vi "Motor controller.vi"(0 "Conveyer Belt":dbl, 1 "Roller":dbl, 2 "Cannon":dbl, 3 "Transfer":dbl, 4 "Flipper":dbl, 5 "Feeder":dbl, 6 "zAvit":dbl, 7 "Camera Servo Y":dbl, 8 "Camera Servo X":dbl, 9 "Canenet":dbl, 10 "Climb Telescopic":dbl) -> ()   [LabVIEW 2012]
uses:
  BotStatus.vi
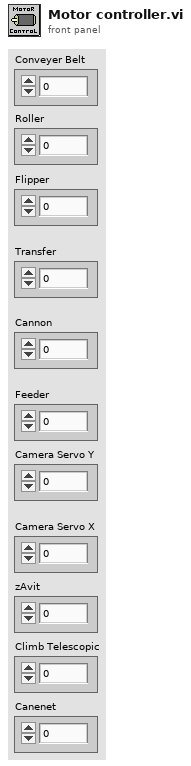
[diagram p1: front panel]
types:
  T1 = typedef "WPI_MotorControlDeviceRef.ctl" = cluster{"DeviceStatus":errorcluster, "Type":enum16{"PWM", "CAN"}, "PWM":cluster{"Digital Module":T2, "PWM Channel":T3, "DeadBand":T4}, "CAN":cluster{"Device Number":u8, "Control Mode":T5, "Semaphore":T6, "Max Vout":dbl}, "Invert":bool, "TransformRef":T7, "InvTransformRef":T7}
  T2 = typedef "FPGA_TypedefDigitalModule.ctl" = enum16{"Digital Module 1", "Digital Module 2"}
  T3 = typedef "FPGA_DIOPWMChannel.ctl" = enum8{"PWM 1", "PWM 2", "PWM 3", "PWM 4", "PWM 5", "PWM 6", "PWM 7", "PWM 8", "PWM 9", "PWM 10", "Invalid"}
  T4 = typedef "WPI_PWMDeadband.ctl" = cluster{"Name":string, "maxPositivePwm":i32, "minPositivePwm":i32, "centerPwm":i32, "maxNegativePwm":i32, "minNegativePwm":i32, "angularRange":u16}
  T5 = typedef "WPI_CANJaguar_ControlMode.ctl" = enum8{"Percent VBus", "Current", "Speed", "Position", "Voltage"}
  T6 = typedef "Semaphore RefNum" = refnum<k1>
  T7 = typedef "WPI_PWMTransform_ConPane.ctl" = refnum<vi>
  T8 = typedef "WPI_ServoDeviceRef.ctl" = cluster{"DeviceStatus":errorcluster, "Digital Module":T2, "PWM Channel":T3, "DeadBand":T4}
  T9 = typedef "WPI_RelayDevRef.ctl" = cluster{"DevStatus":errorcluster, "Relay Channel":T10, "Digital Module":T2, "Relay Direction":T11}
  T10 = typedef "FPGA_DIORelayChannel.ctl" = enum8{"Relay 1", "Relay 2", "Relay 3", "Relay 4", "Relay 5", "Relay 6", "Relay 7", "Relay 8", "Invalid"}
  T11 = typedef "WPI_RelayDirection.ctl" = enum16{"Both directions", "Forward only", "Reverse only"}
  T12 = typedef "WPI_RelayValue.ctl" = enum16{"Off", "On", "Forward", "Reverse"}
  T13 = cluster{"Cannon Upper LS":bool, "Cannon Lower LS":bool}
  T14 = typedef "WPI_DigitalInputDevRef.ctl" = cluster{"DevStatus":errorcluster, "DIO Channel":T15, "Digital Module":T2}
  T15 = typedef "FPGA_DIOChannel.ctl" = enum8{"DIO 1", "DIO 2", "DIO 3", "DIO 4", "DIO 5", "DIO 6", "DIO 7", "DIO 8", "DIO 9", "DIO 10", "DIO 11", "DIO 12", "DIO 13", "DIO 14", "Invalid"}
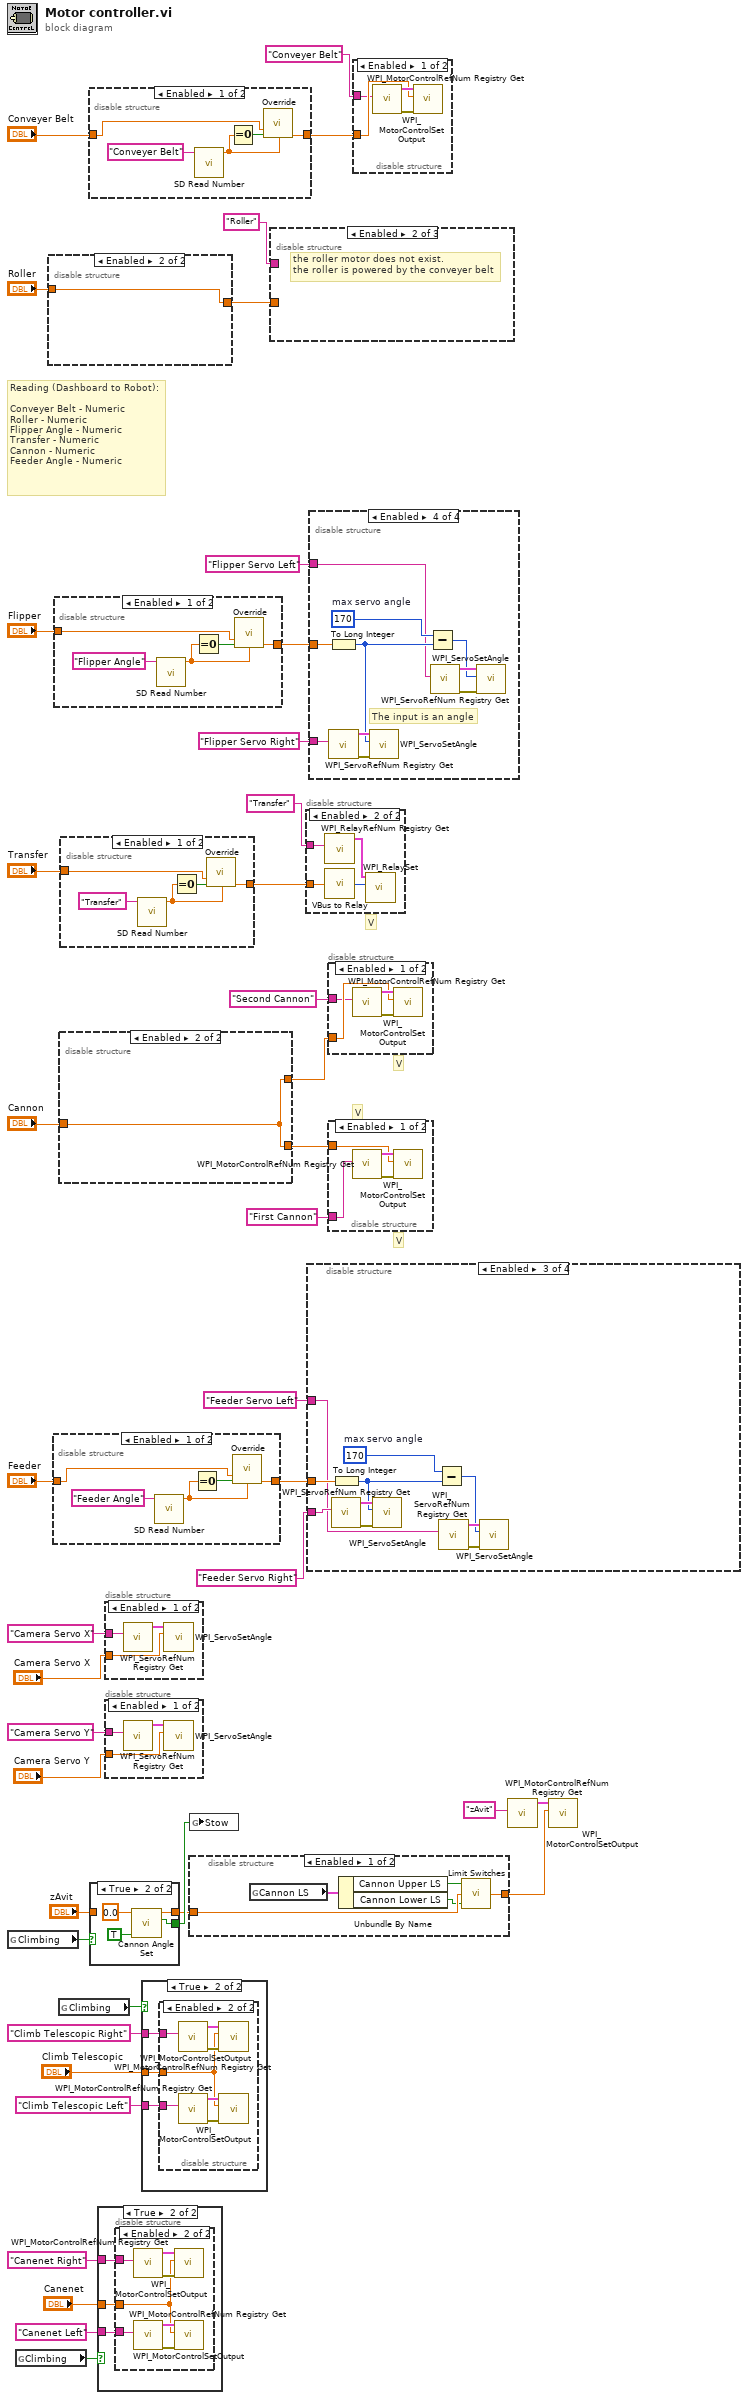
[diagram p0: block diagram]
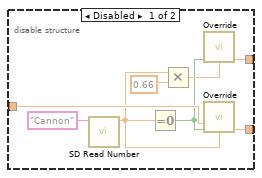
[diagram p5: hidden frame]
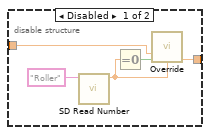
[diagram p8: hidden frame]
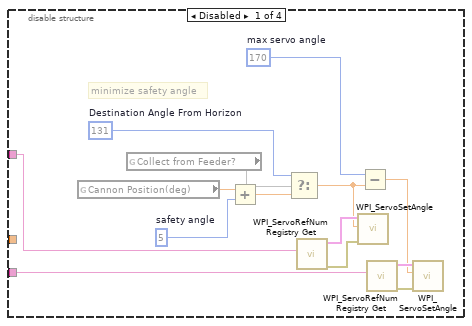
[diagram p11: hidden frame]
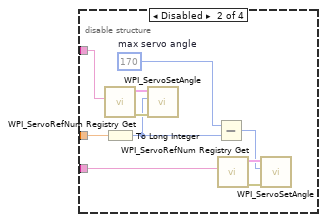
[diagram p12: hidden frame]
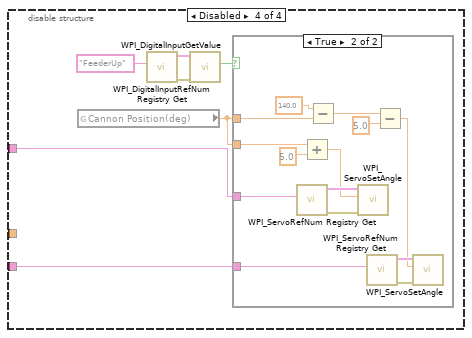
[diagram p13: hidden frame]
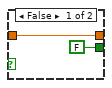
[diagram p15: hidden frame]
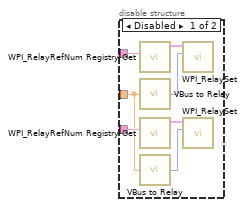
[diagram p19: hidden frame]
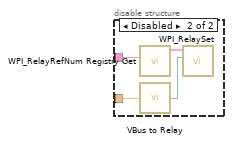
[diagram p20: hidden frame]
diagram:
  # "Reading (Dashboard to Robot):\n\nConveyer Belt - Numeric\nRoller - Numeric\nFlipper Angle - Numeric\nTransfer - Numeric\nCannon - Numeric\nFeeder Angle - Numeric"
  # "V"
  # "V"
  # "V"
  # "V"
  n1 = global read "BotStatus.vi" "Climbing"() -> (w27:bool)
  n2 = global read "BotStatus.vi" "Climbing"() -> (w28:bool)
  n3 = disable-structure shown="Enabled" {
    disable-tunnel: "Roller" -> [w43 w47]
    disable-tunnel: [w42 w47] -> w20
    frame Disabled {
      n4 = call <vilib>:"SD Read Number.vi"("Name"="Roller") -> ("Numeric"=w45:dbl)  [unwired: 8 in, 2 out]
      n5 = Equal To 0?(x=w45) -> (x = 0?=w46:bool)
      n6 = call "Override.vi"("Regualer"=w43, "Override"=w46, "Overriden"=w45) -> ("Output"=w42:dbl)  [unwired: 12 in]
    }
    frame Enabled {
    }
  }
  n7 = disable-structure shown="Enabled" {
    disable-tunnel: [w49 w53] -> w15
    disable-tunnel: "Feeder" -> [w48 w53]
    frame Enabled {
      n8 = call <vilib>:"SD Read Number.vi"("Name"="Feeder Angle") -> ("Numeric"=w52:dbl)  [unwired: 8 in, 2 out]
      n9 = Equal To 0?(x=w52) -> (x = 0?=w51:bool)
      n10 = call "Override.vi"("Regualer"=w48, "Override"=w51, "Overriden"=w52) -> ("Output"=w49:dbl)  [unwired: 12 in]
    }
    frame Disabled {
    }
  }
  n11 = disable-structure shown="Enabled" {
    disable-tunnel: "Flipper" -> [w55 w59]
    disable-tunnel: [w54 w59] -> w19
    frame Enabled {
      n12 = call <vilib>:"SD Read Number.vi"("Name"="Flipper Angle") -> ("Numeric"=w57:dbl)  [unwired: 8 in, 2 out]
      n13 = Equal To 0?(x=w57) -> (x = 0?=w56:bool)
      n14 = call "Override.vi"("Regualer"=w55, "Override"=w56, "Overriden"=w57) -> ("Output"=w54:dbl)  [unwired: 12 in]
    }
    frame Disabled {
    }
  }
  n15 = global read "BotStatus.vi" "Climbing"() -> (w33:bool)
  n16 = disable-structure shown="Enabled" {
    disable-tunnel: "Cannon" -> [w66 w68]
    disable-tunnel: [w65 w68] -> w17
    disable-tunnel: [w60 w68] -> w16
    frame Disabled {
      n17 = call <vilib>:"SD Read Number.vi"("Name"="Cannon") -> ("Numeric"=w63:dbl)  [unwired: 8 in, 2 out]
      n18 = Equal To 0?(x=w63) -> (x = 0?=w64:bool)
      n19 = Multiply(x=w63, y=0.66) -> (x*y=w62:dbl)
      n20 = call "Override.vi"("Override"=w64, "Overriden"=w62) -> ("Output"=w60:dbl)  [unwired: 13 in]
      n21 = call "Override.vi"("Regualer"=w66, "Override"=w64, "Overriden"=w63) -> ("Output"=w65:dbl)  [unwired: 12 in]
    }
    frame Enabled {
    }
  }
  n22 = disable-structure shown="Enabled" {
    disable-tunnel: "Transfer" -> [w70 w74]
    disable-tunnel: [w69 w74] -> w18
    frame Enabled {
      n23 = call <vilib>:"SD Read Number.vi"("Name"="Transfer") -> ("Numeric"=w72:dbl)  [unwired: 8 in, 2 out]
      n24 = Equal To 0?(x=w72) -> (x = 0?=w71:bool)
      n25 = call "Override.vi"("Regualer"=w70, "Override"=w71, "Overriden"=w72) -> ("Output"=w69:dbl)  [unwired: 12 in]
    }
    frame Disabled {
    }
  }
  n26 = disable-structure shown="Enabled" {
    disable-tunnel: [w79 w80] -> w21
    disable-tunnel: "Conveyer Belt" -> [w76 w80]
    frame Enabled {
      n27 = call <vilib>:"SD Read Number.vi"("Name"="Conveyer Belt") -> ("Numeric"=w77:dbl)  [unwired: 8 in, 2 out]
      n28 = Equal To 0?(x=w77) -> (x = 0?=w75:bool)
      n29 = call "Override.vi"("Regualer"=w76, "Override"=w75, "Overriden"=w77) -> ("Output"=w79:dbl)  [unwired: 12 in]
    }
    frame Disabled {
    }
  }
  n30 = case shown="True" w27 {
    tunnel: [w82 w84] -> w14
    tunnel: "zAvit" -> [w82 _]
    tunnel: [FALSE ("On Target") w83] -> w23
    frame False {
    }
    frame True {
      n31 = call "Cannon Angle Set.vi"("set angle 0 to be min angle"=TRUE, "Angle Set Point"=0.0) -> ("On Target"=w83:bool, "zAvit Vbus Out"=w84:dbl)  [unwired: 8 in]
    }
  }
  n32 = case shown="True" w28 {
    tunnel: "Canenet" -> [_ w89]
    tunnel: "Canenet Right" ("refnum name") -> [_ w88]
    tunnel: "Canenet Left" ("refnum name") -> [_ w87]
    frame False {
    }
    frame True {
      n33 = disable-structure shown="Enabled" {
        disable-tunnel: w89 -> [_ w90]
        disable-tunnel: w88 -> [_ w92]
        disable-tunnel: w87 -> [_ w91]
        frame Disabled {
        }
        frame Enabled {
          n34 = call <vilib>:"WPI_MotorControlRefNum Registry Get.vi"("refnum name"=w92) -> ("error out"=w96:errorcluster, "MotorControlDevRef"=w95:T1)  [unwired: 9 in]
          n35 = call <vilib>:"WPI_MotorControlRefNum Registry Get.vi"("refnum name"=w91) -> ("error out"=w93:errorcluster, "MotorControlDevRef"=w94:T1)  [unwired: 9 in]
          n36 = call <vilib>:"WPI_MotorControlSetOutput.vi"("error in (no error)"=w96, "Output"=w90, "MotorControlDevRef"=w95) -> ()  [unwired: 6 in, 3 out]
          n37 = call <vilib>:"WPI_MotorControlSetOutput.vi"("error in (no error)"=w93, "Output"=w90, "MotorControlDevRef"=w94) -> ()  [unwired: 6 in, 3 out]
        }
      }
    }
  }
  n38 = disable-structure shown="Enabled" {
    disable-tunnel: "Camera Servo X" ("refnum name") -> [w99 _]
    disable-tunnel: "Camera Servo X" -> [w97 _]
    frame Enabled {
      n39 = call <vilib>:"WPI_ServoRefNum Registry Get.vi"("refnum name"=w99) -> ("ServoDeviceRef"=w98:T8)  [unwired: 9 in, 1 out]
      n40 = call <vilib>:"WPI_ServoSetAngle.vi"("Angle"=w97, "ServoDeviceRef"=w98) -> ()  [unwired: 8 in, 2 out]
    }
    frame Disabled {
    }
  }
  n41 = disable-structure shown="Enabled" {
    disable-tunnel: "Camera Servo Y" ("refnum name") -> [w102 _]
    disable-tunnel: "Camera Servo Y" -> [w100 _]
    frame Enabled {
      n42 = call <vilib>:"WPI_ServoRefNum Registry Get.vi"("refnum name"=w102) -> ("ServoDeviceRef"=w101:T8)  [unwired: 9 in, 1 out]
      n43 = call <vilib>:"WPI_ServoSetAngle.vi"("Angle"=w100, "ServoDeviceRef"=w101) -> ()  [unwired: 8 in, 2 out]
    }
    frame Disabled {
    }
  }
  n44 = case shown="True" w33 {
    tunnel: "Climb Telescopic" -> [_ w105]
    tunnel: "Climb Telescopic Right" ("refnum name") -> [_ w104]
    tunnel: "Climb Telescopic Left" ("refnum name") -> [_ w103]
    frame False {
    }
    frame True {
      n45 = disable-structure shown="Enabled" {
        disable-tunnel: w105 -> [w107 w113]
        disable-tunnel: w104 -> [w108 w115]
        disable-tunnel: w103 -> [w109 w114]
        frame Disabled {
          n46 = call <vilib>:"WPI_RelayRefNum Registry Get.vi"("refnum name"=w108) -> ("RelayDevRef"=w106:T9)  [unwired: 9 in, 1 out]
          n47 = call "VBus to Relay.vi"("Motor VBus"=w107) -> ("RelayValue"=w112:T12)  [unwired: 3 in]
          n48 = call <vilib>:"WPI_RelayRefNum Registry Get.vi"("refnum name"=w109) -> ("RelayDevRef"=w111:T9)  [unwired: 9 in, 1 out]
          n49 = call "VBus to Relay.vi"("Motor VBus"=w107) -> ("RelayValue"=w110:T12)  [unwired: 3 in]
          n50 = call <vilib>:"WPI_RelaySet.vi"("RelayValue"=w112, "RelayDevRef"=w106) -> ()  [unwired: 8 in, 2 out]
          n51 = call <vilib>:"WPI_RelaySet.vi"("RelayValue"=w110, "RelayDevRef"=w111) -> ()  [unwired: 8 in, 2 out]
        }
        frame Enabled {
          n52 = call <vilib>:"WPI_MotorControlRefNum Registry Get.vi"("refnum name"=w115) -> ("error out"=w119:errorcluster, "MotorControlDevRef"=w118:T1)  [unwired: 9 in]
          n53 = call <vilib>:"WPI_MotorControlRefNum Registry Get.vi"("refnum name"=w114) -> ("error out"=w116:errorcluster, "MotorControlDevRef"=w117:T1)  [unwired: 9 in]
          n54 = call <vilib>:"WPI_MotorControlSetOutput.vi"("error in (no error)"=w119, "Output"=w113, "MotorControlDevRef"=w118) -> ()  [unwired: 6 in, 3 out]
          n55 = call <vilib>:"WPI_MotorControlSetOutput.vi"("error in (no error)"=w116, "Output"=w113, "MotorControlDevRef"=w117) -> ()  [unwired: 6 in, 3 out]
        }
      }
    }
  }
  n56 = global write "BotStatus.vi" "Stow"(w23) -> ()
  n57 = disable-structure shown="Enabled" {
    disable-tunnel: w14 -> [w123 w125]
    disable-tunnel: [w124 w125] -> w13
    frame Enabled {
      n58 = global read "BotStatus.vi" "Cannon LS"() -> (w122:T13)
      n59 = Unbundle By Name(w122) -> ("Cannon Upper LS"=w121:bool, "Cannon Lower LS"=w120:bool)
      n60 = call "Limit Switches.vi"("Backward Limit Switch"=w120, "VBus in"=w123, "Forward Limit Switch"=w121) -> ("VBus out"=w124:dbl)
    }
    frame Disabled {
    }
  }
  n61 = disable-structure shown="Enabled" {
    disable-tunnel: w20 -> [w127 _ w130]
    disable-tunnel: "Roller" ("refnum name") -> [w126 _ w132]
    frame Disabled {
      n62 = call <vilib>:"WPI_MotorControlRefNum Registry Get.vi"("refnum name"=w126) -> ("error out"=w129:errorcluster, "MotorControlDevRef"=w128:T1)  [unwired: 9 in]
      n63 = call <vilib>:"WPI_MotorControlSetOutput.vi"("error in (no error)"=w129, "Output"=w127, "MotorControlDevRef"=w128) -> ()  [unwired: 6 in, 3 out]
    }
    frame Enabled {
      # "the roller motor does not exist.\nthe roller is powered by the conveyer belt"
    }
    frame Disabled {
      n64 = call <vilib>:"WPI_RelayRefNum Registry Get.vi"("refnum name"=w132) -> ("RelayDevRef"=w131:T9)  [unwired: 9 in, 1 out]
      n65 = call "VBus to Relay.vi"("Motor VBus"=w130) -> ("RelayValue"=w133:T12)  [unwired: 3 in]
      n66 = call <vilib>:"WPI_RelaySet.vi"("RelayValue"=w133, "RelayDevRef"=w131) -> ()  [unwired: 8 in, 2 out]
    }
  }
  n67 = disable-structure shown="Enabled" {
    disable-tunnel: w18 -> [w135 w138]
    disable-tunnel: "Transfer" ("refnum name") -> [w134 w140]
    frame Disabled {
      n68 = call <vilib>:"WPI_MotorControlRefNum Registry Get.vi"("refnum name"=w134) -> ("error out"=w137:errorcluster, "MotorControlDevRef"=w136:T1)  [unwired: 9 in]
      n69 = call <vilib>:"WPI_MotorControlSetOutput.vi"("error in (no error)"=w137, "Output"=w135, "MotorControlDevRef"=w136) -> ()  [unwired: 6 in, 3 out]
    }
    frame Enabled {
      n70 = call <vilib>:"WPI_RelayRefNum Registry Get.vi"("refnum name"=w140) -> ("RelayDevRef"=w139:T9)  [unwired: 9 in, 1 out]
      n71 = call "VBus to Relay.vi"("Motor VBus"=w138) -> ("RelayValue"=w141:T12)  [unwired: 3 in]
      n72 = call <vilib>:"WPI_RelaySet.vi"("RelayValue"=w141, "RelayDevRef"=w139) -> ()  [unwired: 8 in, 2 out]
    }
  }
  n73 = disable-structure shown="Enabled" {
    disable-tunnel: "Feeder Servo Left" ("refnum name") -> [w152 w157 w166 w178]
    disable-tunnel: "Feeder Servo Right" ("refnum name") -> [w149 w156 w167 w177]
    disable-tunnel: w15 -> [_ w159 w169 _]
    frame Disabled {
      w144 = 131  # Destination Angle From Horizon
      w148 = 170  # max servo angle
      w153 = 5  # safety angle
      # "minimize safety angle"
      n74 = global read "BotStatus.vi" "Cannon Position(deg)"() -> (w142:dbl)
      n75 = global read "BotStatus.vi" "Collect from Feeder?"() -> (w143)
      n76 = Add(x=w142, y=w153) -> (x+y=w145:dbl)
      n77 = Select(t=w144, s=w143, f=w145) -> (s? t:f=w146:dbl)
      n78 = call <vilib>:"WPI_ServoRefNum Registry Get.vi"("refnum name"=w152) -> ("error out"=w154:errorcluster, "ServoDeviceRef"=w155:T8)  [unwired: 9 in]
      n79 = call <vilib>:"WPI_ServoSetAngle.vi"("error in (no error)"=w154, "Angle"=w146, "ServoDeviceRef"=w155) -> ()  [unwired: 7 in, 2 out]
      n80 = Subtract(x=w148, y=w146) -> (x-y=w147:dbl)
      n81 = call <vilib>:"WPI_ServoRefNum Registry Get.vi"("refnum name"=w149) -> ("error out"=w150:errorcluster, "ServoDeviceRef"=w151:T8)  [unwired: 9 in]
      n82 = call <vilib>:"WPI_ServoSetAngle.vi"("error in (no error)"=w150, "Angle"=w147, "ServoDeviceRef"=w151) -> ()  [unwired: 7 in, 2 out]
    }
    frame Disabled {
      w161 = 170  # max servo angle
      n83 = call <vilib>:"WPI_ServoRefNum Registry Get.vi"("refnum name"=w157) -> ("error out"=w164:errorcluster, "ServoDeviceRef"=w165:T8)  [unwired: 9 in]
      n84 = To Long Integer(number=w159) -> (32bit integer=w158:i32)
      n85 = call <vilib>:"WPI_ServoSetAngle.vi"("error in (no error)"=w164, "Angle"=w158, "ServoDeviceRef"=w165) -> ()  [unwired: 7 in, 2 out]
      n86 = Subtract(x=w161, y=w158) -> (x-y=w160:i32)
      n87 = call <vilib>:"WPI_ServoRefNum Registry Get.vi"("refnum name"=w156) -> ("error out"=w162:errorcluster, "ServoDeviceRef"=w163:T8)  [unwired: 9 in]
      n88 = call <vilib>:"WPI_ServoSetAngle.vi"("error in (no error)"=w162, "Angle"=w160, "ServoDeviceRef"=w163) -> ()  [unwired: 7 in, 2 out]
    }
    frame Enabled {
      w171 = 170  # max servo angle
      n89 = To Long Integer(number=w169) -> (32bit integer=w168:i32)
      n90 = call <vilib>:"WPI_ServoRefNum Registry Get.vi"("refnum name"=w167) -> ("error out"=w174:errorcluster, "ServoDeviceRef"=w175:T8)  [unwired: 9 in]
      n91 = call <vilib>:"WPI_ServoSetAngle.vi"("error in (no error)"=w174, "Angle"=w168, "ServoDeviceRef"=w175) -> ()  [unwired: 7 in, 2 out]
      n92 = Subtract(x=w171, y=w168) -> (x-y=w170:i32)
      n93 = call <vilib>:"WPI_ServoRefNum Registry Get.vi"("refnum name"=w166) -> ("error out"=w172:errorcluster, "ServoDeviceRef"=w173:T8)  [unwired: 9 in]
      n94 = call <vilib>:"WPI_ServoSetAngle.vi"("error in (no error)"=w172, "Angle"=w170, "ServoDeviceRef"=w173) -> ()  [unwired: 7 in, 2 out]
    }
    frame Disabled {
      n95 = global read "BotStatus.vi" "Cannon Position(deg)"() -> (w176:dbl)
      n96 = call <vilib>:"WPI_DigitalInputRefNum Registry Get.vi"("refnum name"="FeederUp") -> ("error out"=w180:errorcluster, "DigitalInputDevRef"=w179:T14)  [unwired: 9 in]
      n97 = call <vilib>:"WPI_DigitalInputGetValue.vi"("error in (no error)"=w180, "DigitalInputDevRef"=w179) -> ("Value"=w182:bool)  [unwired: 7 in, 2 out]
      n98 = case shown="True" w182 {
        tunnel: w178 -> [_ w194]
        tunnel: w176 -> [_ w193]
        tunnel: w177 -> [_ w185]
        tunnel: w176 -> [_ w184]
        frame False {
        }
        frame True {
          n99 = call <vilib>:"WPI_ServoRefNum Registry Get.vi"("refnum name"=w194) -> ("error out"=w195:errorcluster, "ServoDeviceRef"=w196:T8)  [unwired: 9 in]
          n100 = Add(x=w193, y=5.0) -> (x+y=w191:dbl)
          n101 = Subtract(x=140.0, y=w184) -> (x-y=w189:dbl)
          n102 = call <vilib>:"WPI_ServoSetAngle.vi"("error in (no error)"=w195, "Angle"=w191, "ServoDeviceRef"=w196) -> ()  [unwired: 7 in, 2 out]
          n103 = call <vilib>:"WPI_ServoRefNum Registry Get.vi"("refnum name"=w185) -> ("error out"=w186:errorcluster, "ServoDeviceRef"=w187:T8)  [unwired: 9 in]
          n104 = Subtract(x=w189, y=5.0) -> (x-y=w183:dbl)
          n105 = call <vilib>:"WPI_ServoSetAngle.vi"("error in (no error)"=w186, "Angle"=w183, "ServoDeviceRef"=w187) -> ()  [unwired: 7 in, 2 out]
        }
      }
    }
  }
  n106 = disable-structure shown="Enabled" {
    disable-tunnel: w19 -> [w198 w201 w211 w222]
    disable-tunnel: "Flipper Servo Left" ("refnum name") -> [w197 w203 w214 w216]
    disable-tunnel: "Flipper Servo Right" ("refnum name") -> [_ _ w205 w215]
    frame Disabled {
      n107 = call <vilib>:"WPI_MotorControlRefNum Registry Get.vi"("refnum name"=w197) -> ("error out"=w200:errorcluster, "MotorControlDevRef"=w199:T1)  [unwired: 9 in]
      n108 = call <vilib>:"WPI_MotorControlSetOutput.vi"("error in (no error)"=w200, "Output"=w198, "MotorControlDevRef"=w199) -> ()  [unwired: 6 in, 3 out]
    }
    frame Disabled {
      n109 = call <vilib>:"WPI_RelayRefNum Registry Get.vi"("refnum name"=w203) -> ("RelayDevRef"=w202:T9)  [unwired: 9 in, 1 out]
      n110 = call "VBus to Relay.vi"("Motor VBus"=w201) -> ("RelayValue"=w204:T12)  [unwired: 3 in]
      n111 = call <vilib>:"WPI_RelaySet.vi"("RelayValue"=w204, "RelayDevRef"=w202) -> ()  [unwired: 8 in, 2 out]
    }
    frame Disabled {
      w208 = 170  # max servo angle
      # "The input is an angle"
      n112 = call <vilib>:"WPI_ServoRefNum Registry Get.vi"("refnum name"=w214) -> ("error out"=w212:errorcluster, "ServoDeviceRef"=w213:T8)  [unwired: 9 in]
      n113 = To Long Integer(number=w211) -> (32bit integer=w207:i32)
      n114 = call <vilib>:"WPI_ServoSetAngle.vi"("error in (no error)"=w212, "Angle"=w207, "ServoDeviceRef"=w213) -> ()  [unwired: 7 in, 2 out]
      n115 = Subtract(x=w208, y=w207) -> (x-y=w206:i32)
      n116 = call <vilib>:"WPI_ServoRefNum Registry Get.vi"("refnum name"=w205) -> ("error out"=w210:errorcluster, "ServoDeviceRef"=w209:T8)  [unwired: 9 in]
      n117 = call <vilib>:"WPI_ServoSetAngle.vi"("error in (no error)"=w210, "Angle"=w206, "ServoDeviceRef"=w209) -> ()  [unwired: 7 in, 2 out]
    }
    frame Enabled {
      w219 = 170  # max servo angle
      # "The input is an angle"
      n118 = To Long Integer(number=w222) -> (32bit integer=w218:i32)
      n119 = call <vilib>:"WPI_ServoRefNum Registry Get.vi"("refnum name"=w215) -> ("error out"=w223:errorcluster, "ServoDeviceRef"=w224:T8)  [unwired: 9 in]
      n120 = call <vilib>:"WPI_ServoSetAngle.vi"("error in (no error)"=w223, "Angle"=w218, "ServoDeviceRef"=w224) -> ()  [unwired: 7 in, 2 out]
      n121 = Subtract(x=w219, y=w218) -> (x-y=w217:i32)
      n122 = call <vilib>:"WPI_ServoRefNum Registry Get.vi"("refnum name"=w216) -> ("error out"=w221:errorcluster, "ServoDeviceRef"=w220:T8)  [unwired: 9 in]
      n123 = call <vilib>:"WPI_ServoSetAngle.vi"("error in (no error)"=w221, "Angle"=w217, "ServoDeviceRef"=w220) -> ()  [unwired: 7 in, 2 out]
    }
  }
  n124 = disable-structure shown="Enabled" {
    disable-tunnel: w16 -> [w226 w229]
    disable-tunnel: "Second Cannon" ("refnum name") -> [w225 w231]
    frame Enabled {
      n125 = call <vilib>:"WPI_MotorControlRefNum Registry Get.vi"("refnum name"=w225) -> ("error out"=w228:errorcluster, "MotorControlDevRef"=w227:T1)  [unwired: 9 in]
      n126 = call <vilib>:"WPI_MotorControlSetOutput.vi"("error in (no error)"=w228, "Output"=w226, "MotorControlDevRef"=w227) -> ()  [unwired: 6 in, 3 out]
    }
    frame Disabled {
      n127 = call <vilib>:"WPI_RelayRefNum Registry Get.vi"("refnum name"=w231) -> ("RelayDevRef"=w230:T9)  [unwired: 9 in, 1 out]
      n128 = call "VBus to Relay.vi"("Motor VBus"=w229) -> ("RelayValue"=w232:T12)  [unwired: 3 in]
      n129 = call <vilib>:"WPI_RelaySet.vi"("RelayValue"=w232, "RelayDevRef"=w230) -> ()  [unwired: 8 in, 2 out]
    }
  }
  n130 = disable-structure shown="Enabled" {
    disable-tunnel: w17 -> [w234 w237]
    disable-tunnel: "First Cannon" ("refnum name") -> [w233 w239]
    frame Enabled {
      n131 = call <vilib>:"WPI_MotorControlRefNum Registry Get.vi"("refnum name"=w233) -> ("error out"=w236:errorcluster, "MotorControlDevRef"=w235:T1)  [unwired: 9 in]
      n132 = call <vilib>:"WPI_MotorControlSetOutput.vi"("error in (no error)"=w236, "Output"=w234, "MotorControlDevRef"=w235) -> ()  [unwired: 6 in, 3 out]
    }
    frame Disabled {
      n133 = call <vilib>:"WPI_RelayRefNum Registry Get.vi"("refnum name"=w239) -> ("RelayDevRef"=w238:T9)  [unwired: 9 in, 1 out]
      n134 = call "VBus to Relay.vi"("Motor VBus"=w237) -> ("RelayValue"=w240:T12)  [unwired: 3 in]
      n135 = call <vilib>:"WPI_RelaySet.vi"("RelayValue"=w240, "RelayDevRef"=w238) -> ()  [unwired: 8 in, 2 out]
    }
  }
  n136 = disable-structure shown="Enabled" {
    disable-tunnel: w21 -> [w242 w245]
    disable-tunnel: "Conveyer Belt" ("refnum name") -> [w241 w247]
    frame Enabled {
      n137 = call <vilib>:"WPI_MotorControlRefNum Registry Get.vi"("refnum name"=w241) -> ("error out"=w244:errorcluster, "MotorControlDevRef"=w243:T1)  [unwired: 9 in]
      n138 = call <vilib>:"WPI_MotorControlSetOutput.vi"("error in (no error)"=w244, "Output"=w242, "MotorControlDevRef"=w243) -> ()  [unwired: 6 in, 3 out]
    }
    frame Disabled {
      n139 = call <vilib>:"WPI_RelayRefNum Registry Get.vi"("refnum name"=w247) -> ("RelayDevRef"=w246:T9)  [unwired: 9 in, 1 out]
      n140 = call "VBus to Relay.vi"("Motor VBus"=w245) -> ("RelayValue"=w248:T12)  [unwired: 3 in]
      n141 = call <vilib>:"WPI_RelaySet.vi"("RelayValue"=w248, "RelayDevRef"=w246) -> ()  [unwired: 8 in, 2 out]
    }
  }
  n142 = call <vilib>:"WPI_MotorControlRefNum Registry Get.vi"("refnum name"="zAvit") -> ("MotorControlDevRef"=w25:T1)  [unwired: 9 in, 1 out]
  n143 = call <vilib>:"WPI_MotorControlSetOutput.vi"("Output"=w13, "MotorControlDevRef"=w25) -> ()  [unwired: 7 in, 3 out]
